vi "Initialize ACS.vi"(8 "error in (no error)":errorcluster, 11 "SPARC4_GEI in":refnum<class "S4GEI.lvclass">) -> (0 "error out":errorcluster, 3 "SPARC4_GEI out":refnum<class "S4GEI.lvclass">)   [LabVIEW 2018, in "S4GEI.lvclass"]
uses:
  S4GEI.lvclass
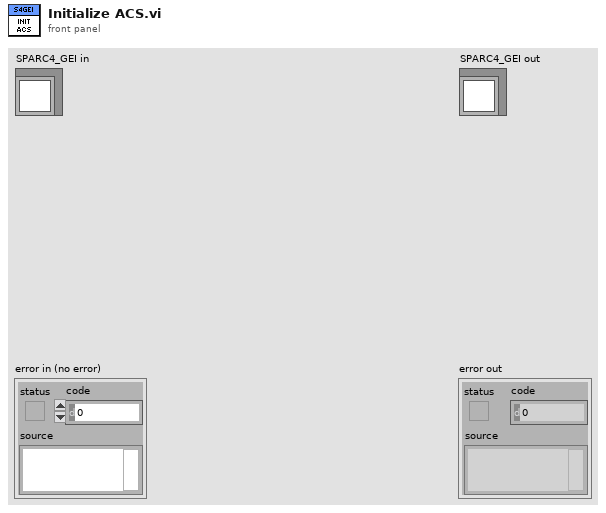
[diagram p1: front panel]
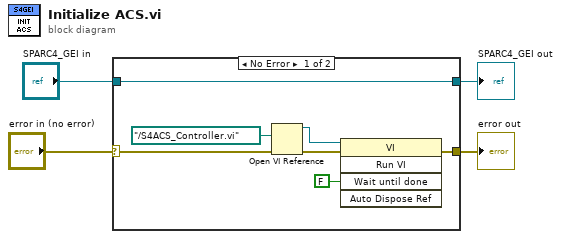
[diagram p0: block diagram]
diagram:
  n1 = case shown="No Error" "error in (no error)" {
    selector: "error in (no error)" -> [w6 w13]
    tunnel: [w5 w13] -> w3
    tunnel: [w11 w12] -> w1
    tunnel: "SPARC4_GEI in" -> [w11 w12]
    frame No Error {
      n2 = Open VI Reference(vi path=path "../S4ACS_Controller.vi", error in (no error)=w6) -> (vi reference=w10:refnum<vi>, error out=w9:errorcluster)  [unwired: 4 in]
      n3 = invoke class="VI" method="Run VI"(reference=w10, error in=w9, "Wait until done"=FALSE ("Wait Until Done")) -> (error out=w5:errorcluster)  [unwired: 2 in, 4 out]
    }
    frame Error {
    }
  }
  "error out" <- w3
  "SPARC4_GEI out" <- w1
